vi "Is Open.vi"(8 "error in (no error)":errorcluster, 11 "SerialResource in":refnum<class "SerialResource.lvclass">) -> (0 "error out":errorcluster, 2 "Is Open":bool, 3 "SerialResource out":refnum<class "SerialResource.lvclass">)   [LabVIEW 2020, in "PicoG-Core.lvlib" / "SerialResource.lvclass"]
uses:
  SerialResource.lvclass
  SerialResource.lvclass/SerialResource.ctl
  <vilib>/IlluminatedG/IG Serial Stream/Stream-Serial/Serial Client/Serial Client.lvclass
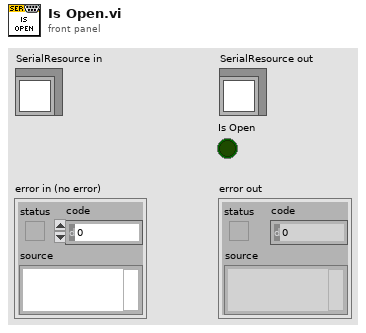
[diagram p1: front panel]
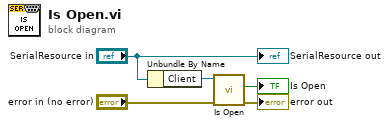
[diagram p0: block diagram]
diagram:
  n1 = Unbundle By Name("SerialResource in") -> ("Client"=w4:refnum<class "Serial Client.lvclass">)
  n2 = call-dynamic "Is Open.vi"("error in (no error)"="error in (no error)", "Serial Client in"=w4) -> ("error out"=→"error out":errorcluster, "Is Open"=→"Is Open":bool)  [unwired: 7 in, 1 out]
  "SerialResource out" <- "SerialResource in"
